vi "ImageMouseWheel.vi"(8 "error in (no error)":errorcluster, 10 "Value":dbl=0.2 format="%#_13g", 11 "Displayer in":refnum<class "Displayer.lvclass">) -> (0 "error out":errorcluster, 3 "Displayer out":refnum<class "Displayer.lvclass">)   [LabVIEW 2020, in "Displayer.lvlib" / "Displayer.lvclass"]
uses:
  Displayer.lvclass
  C:/Program Files/National Instruments/LabVIEW 2020/vi.lib/ActorFramework/Actor/Actor.lvclass
  Model/Hardware Abstraction Layer/Component/Device/Device/DataExchange.ctl
  <vilib>/ActorFramework/Actor/Actor.lvclass/Actor.ctl
  Interface/DataListener Messages/OnDataChange Msg/OnDataChange Msg.lvclass/OnDataChange Msg.ctl
  <vilib>/ActorFramework/Message Enqueuer/Message Enqueuer.lvclass/Message Enqueuer.ctl
  <vilib>/ActorFramework/Message Enqueuer/Enqueue.vi
  Interface/DataListener Messages/OnDataChange Msg/OnDataChange Msg.lvclass
  C:/Program Files/National Instruments/LabVIEW 2020/vi.lib/ActorFramework/Message/Message.lvclass
  <vilib>/ActorFramework/Message Priority Queue/Priority Enqueue.vi
  <vilib>/ActorFramework/Actor/Actor.lvclass
  Interface/DataListener/DataListener.lvclass
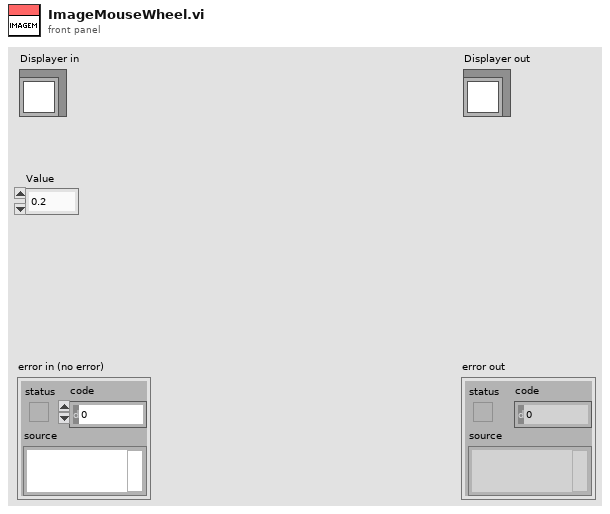
[diagram p1: front panel]
types:
  T1 = typedef "DataListener.lvclass/DataExchange.ctl" = cluster{"Source":string, "Destination":string, "Description":string, "value":variant}
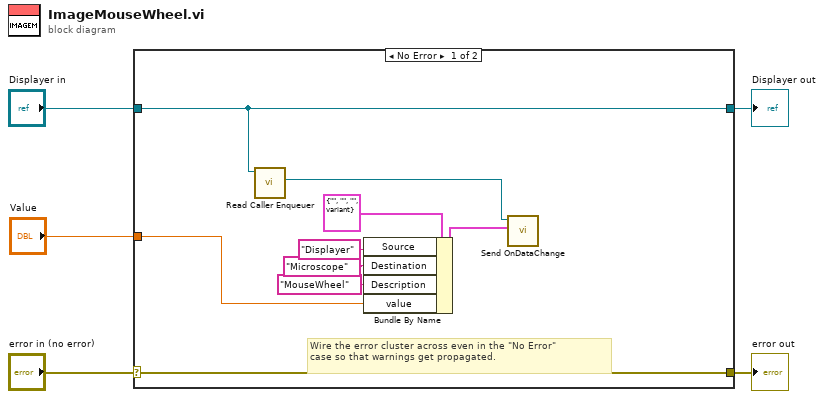
[diagram p0: block diagram]
diagram:
  n1 = case shown="No Error" "error in (no error)" {
    selector: "error in (no error)" -> [w14 w16]
    tunnel: [w14 w16] -> w4
    tunnel: [w13 w15] -> w2
    tunnel: "Displayer in" -> [w13 w15]
    tunnel: "Value" -> [w6 _]
    frame No Error {
      # "Wire the error cluster across even in the \"No Error\"\ncase so that warnings get propagated."
      n2 = call <vilib>:"Read Caller Enqueuer.vi"("Actor"=w13) -> ("Caller Enqueuer"=w12:refnum<class "Message Enqueuer.lvclass">)  [unwired: 10 in]
      n3 = Bundle By Name(cluster=T1 {"Source"="", "Destination"="", "Description"="", "value"=variant} ("DataExchange"), "Source"="Displayer", "Destination"="Microscope", "Description"="MouseWheel", "value"=w6) -> (w10:T1)
      n4 = call "Send OnDataChange.vi"("DataExchange"=w10, "Message Enqueuer"=w12) -> ()  [unwired: 8 in, 2 out]
    }
    frame Error {
    }
  }
  "error out" <- w4
  "Displayer out" <- w2
